vi "fgt get valve range.vi"(8 "error in (no error)":errorcluster, 11 "valveIndex":u32) -> (0 "error out":errorcluster, 3 "max position":i32)   [LabVIEW 2016, in "fgt_SDK.lvlib"]
doc: "Get valve maximum position. Position indexing starts at 0."
uses:
  fgt_SDK.lvlib
  dlls/fgt_SDK_32.dll
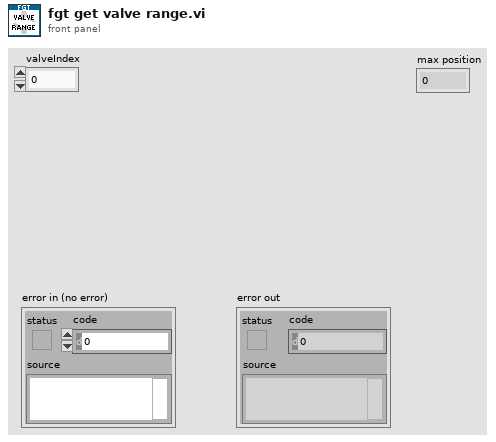
[diagram p1: front panel]
types:
  T1 = typedef "fgt_SDK.lvlib/fgt_STATUS_INFO.ctl" = cluster{"InstrType":T2, "instrSN":u16, "errorCode":u8, "infoCode":u8, "detail":string}
  T2 = typedef "fgt_SDK.lvlib/fgt_INSTRUMENT_TYPE.ctl" = enum32{"None", "MFCS", "MFCS_EZ", "FRP", "LineUP", "IPS", "ESS", "F_OEM"}
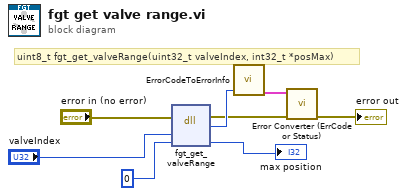
[diagram p0: block diagram]
diagram:
  # "uint8_t fgt_get_valveRange(uint32_t valveIndex, int32_t *posMax)"
  n1 = dll-call lib="C:/projects/SDK/fgt-sdk-labview/dlls/fgt_SDK_*.*" fn="fgt_get_valveRange"(error in="error in (no error)", "valveIndex"="valveIndex", "posMax"=0 ("position")) -> (error out=w4:errorcluster, "return type"=w6:u8, "posMax"=→"max position":i32)  [unwired: 3 in, 1 out]
  n2 = call "ErrorCodeToErrorInfo.vi"("return type"=w6) -> ("StatusInfo"=w5:T1)  [unwired: 10 in]
  n3 = call "Error Converter (ErrCode or Status).vi"("error in (no error)"=w4, "StatusInfo"=w5) -> ("error out"=→"error out":errorcluster)  [unwired: 9 in]
